vi "ITC503controlMonitor.vi"() -> ()   [LabVIEW 2019]
uses:
  Utility/ITC503/ITC503Monitor-Cluster.ctl
  Instrument_Setup.vi
  Global/Global Variables/Data_Display_global.vi
panel:
  out "error out":errorcluster
  in  "error in (no error)":errorcluster
  out "Path":path
  in  "stop":bool
  out "ITC503-Monitor":T1={"Temperatur (K)"=0.0, "Setpoint (K)"=0.0, "Rate (K/min)"=3.4572, "Heater (%)"=0.0, "NV (%)"=0.0, "Heater Manual"=FALSE, "NV Manual"=FALSE, "Go to Set"=FALSE, "Heater SP"=0.0, "Valid?"=FALSE, "Set Heater SP"=FALSE, "Set NV SP"=FALSE, "Heater (%) Display"=3.4572, "NV (%) Display"=3.4572, "NV Setpoint"=0.0, "Change Heater Status"=FALSE, "Change NV Status"=FALSE, "Sample 3"=0.0, "Sample 2"=0.0, "Sweep-State"=FALSE, "Set Auto PID"=FALSE, "Auto PID"=FALSE, "Stopp"=FALSE, "Setpoint-Sweep"=0.0, "Sample 1"=0.0, "Control Channel"=FALSE, "Channel 1"=FALSE, "Channel 2"=FALSE, "Channel 3"=FALSE} {"NV (%) Display" format="%4_5f"; "Heater (%) Display" format="%4_5f"; "NV (%)" scale=0.0..100.0; "Heater (%)" scale=0.0..100.0; "Rate (K/min)" format="%#4_5f"; "Setpoint (K)" format="%6_5f"}
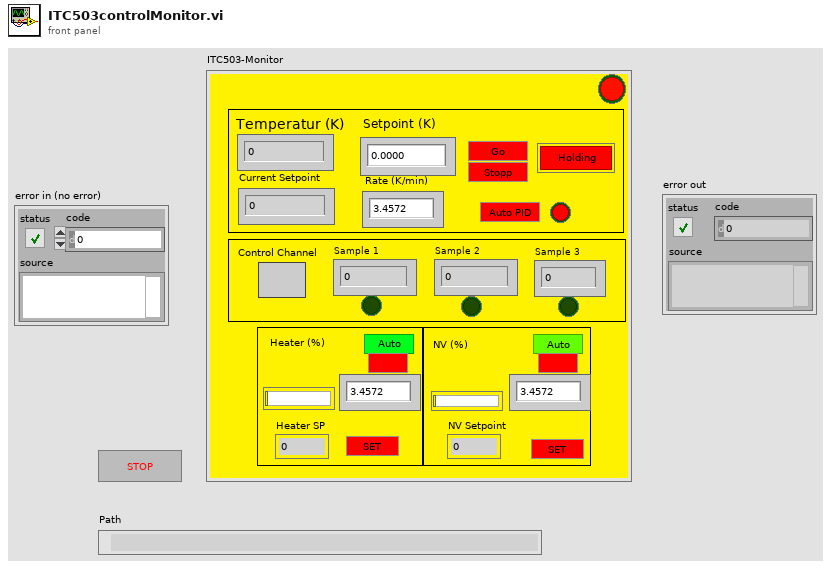
[diagram p1: front panel]
types:
  T1 = typedef "ITC503Monitor-Cluster.ctl" = cluster{"Temperatur (K)":dbl, "Setpoint (K)":dbl, "Rate (K/min)":dbl, "Heater (%)":dbl, "NV (%)":dbl, "Heater Manual":bool, "NV Manual":bool, "Go to Set":bool, "Heater SP":dbl, "Valid?":bool, "Set Heater SP":bool, "Set NV SP":bool, "Heater (%) Display":dbl, "NV (%) Display":dbl, "NV Setpoint":dbl, "Change Heater Status":bool, "Change NV Status":bool, "Sample 3":dbl, "Sample 2":dbl, "Sweep-State":bool, "Set Auto PID":bool, "Auto PID":bool, "Stopp":bool, "Setpoint-Sweep":dbl, "Sample 1":dbl, "Control Channel":bool, "Channel 1":bool, "Channel 2":bool, "Channel 3":bool}
  T2 = cluster{"Com Port":i32, "ISOBUS Address":i32, "GPIB Address":i16, "Communication":enum16{"RS232", "ISOBUS", "GPIB", "Gateway"}}
  T3 = typedef "OxfordAddress.ctl" = cluster{"Com Port":i32, "ISOBUS Address":i32, "GPIB Address":i16, "Communication":enum16{"RS232", "ISOBUS", "GPIB", "Gateway"}}
  T4 = enum32{"Bad", "Idle", "Run top level", "Running"}
  T5 = typedef "ITCIO.ctl" = cluster{"Com Port":i32, "ISOBUS Address":i32, "GPIB Address":i16, "Communication":enum16{"RS232", "ISOBUS", "GPIB", "Gateway"}}
  T6 = typedef "ITC503_control.ctl" = cluster{"Setpoint (K)":dbl, "Rate (K/min)":dbl, "Go to Set":bool, "Set Heater SP":bool, "Set NV SP":bool, "Change Heater Status":bool, "Change NV Status":bool, "Set Auto PID":bool, "Stopp":bool, "Control Channel":bool, "Heater SP":dbl, "NV Setpoint":dbl}
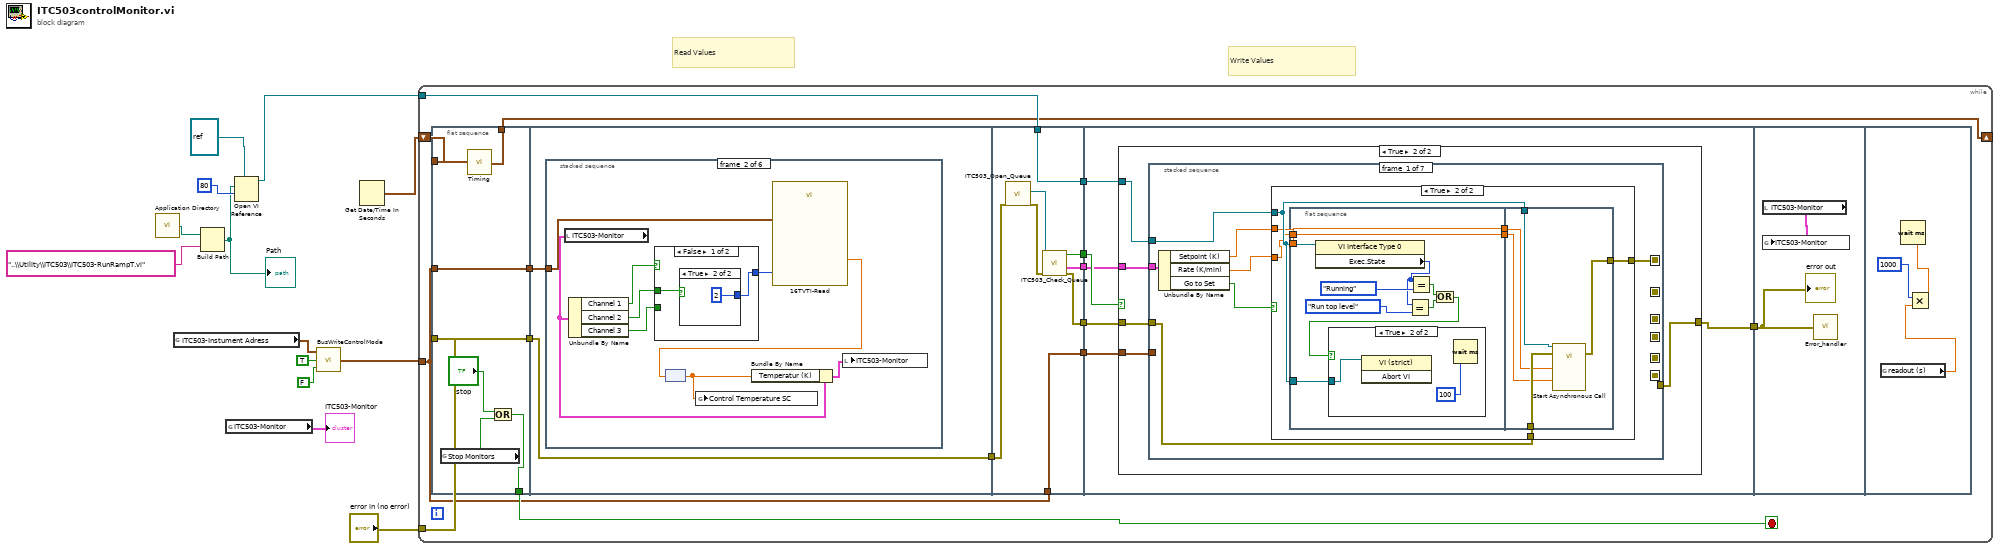
[diagram p0: block diagram]
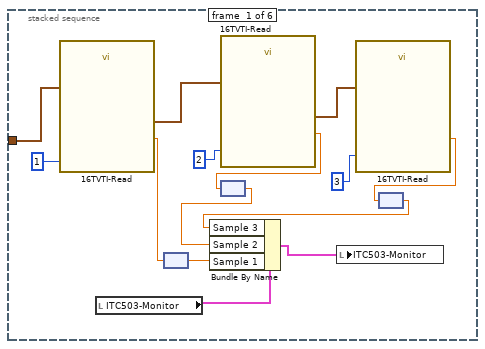
[diagram p2: hidden frame]
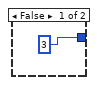
[diagram p3: hidden frame]
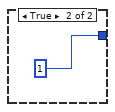
[diagram p4: hidden frame]
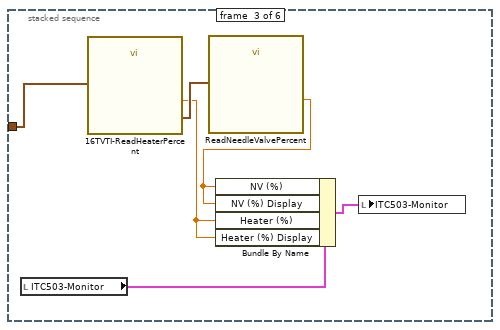
[diagram p5: hidden frame]
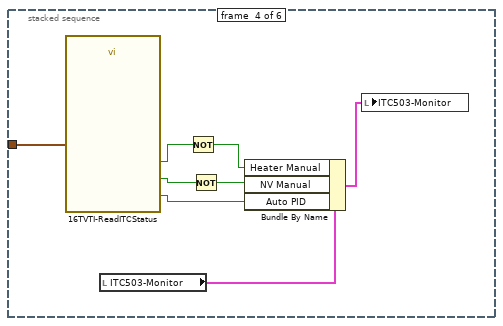
[diagram p6: hidden frame]
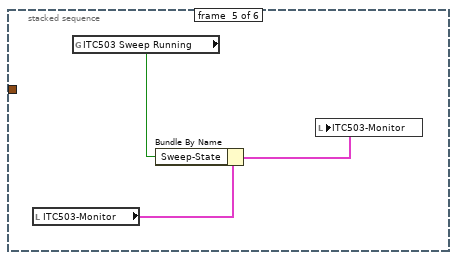
[diagram p7: hidden frame]
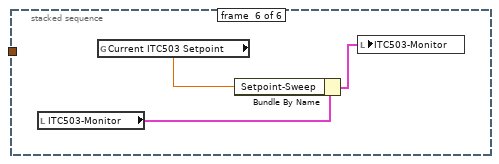
[diagram p8: hidden frame]
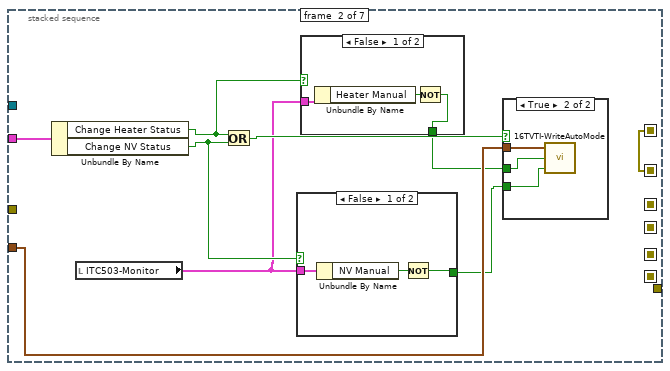
[diagram p12: hidden frame]
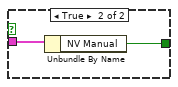
[diagram p14: hidden frame]
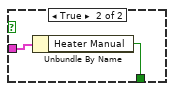
[diagram p15: hidden frame]
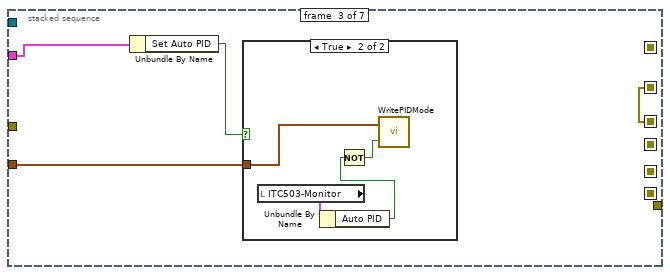
[diagram p16: hidden frame]
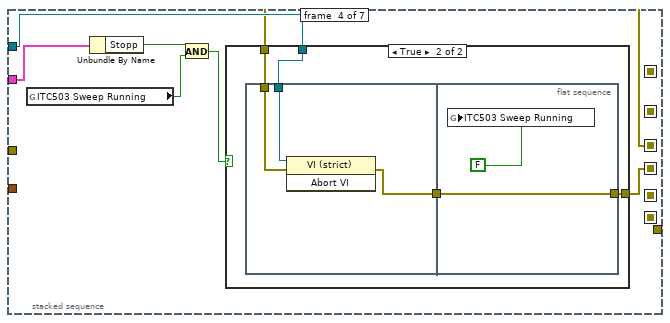
[diagram p18: hidden frame]
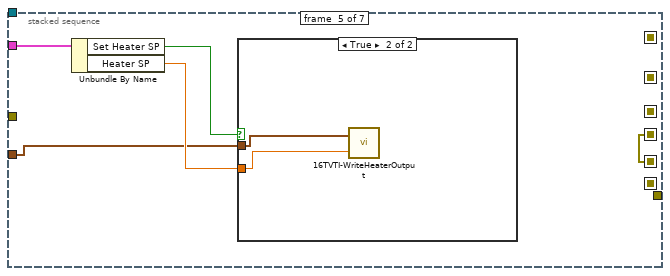
[diagram p20: hidden frame]
diagram:
  # "Write Values"
  # "Read Values"
  n1 = call <vilib>:"Application Directory.vi"() -> ("Application Directory"=w11:path)
  n2 = global read "Instrument_Setup.vi" "ITC503-Instument Adress"() -> (w8:T2)
  n3 = Build Path(base path=w11, name or relative path="..\\Utility\\ITC503\\ITC503-RunRampT.vi") -> (appended path=w9:path)
  "Path" <- w9
  n4 = global read "Data_Display_global.vi" "ITC503-Monitor"() -> (→"ITC503-Monitor":T1)
  n5 = Open VI Reference(type specifier VI Refnum (for type only)=refnum<vi> refnum, vi path=w9, options=80) -> (vi reference=w1:refnum<vi>)  [unwired: 3 in, 1 out]
  n6 = call "BusWriteControlMode.vi"("Locked"=FALSE, "Remote"=TRUE, "Address"=w8) -> ("Address(thru)"=w5:T3)
  n7 = Get Date/Time In Seconds() -> (seconds since 1Jan1904=w3:timestamp)
  n8 = while {
    tunnel: w5 -> [w16]
    shift-right: [w14] -> _
    shift-left: w3 -> [w27]
    tunnel: "error in (no error)" -> [w24]
    tunnel: w1 -> [w17]
    stop <- w28 stop-if-true
    n9 = flat-sequence {
      tunnel: [w33] -> w28
      tunnel: w27 -> [w32]
      tunnel: [w31] -> w14
      tunnel: w16 -> [w30]
      tunnel: [w30] -> w26
      tunnel: [w29] -> w25
      tunnel: w24 -> [w29]
      tunnel: w26 -> [w37]
      tunnel: w25 -> [w36]
      tunnel: [w36] -> w23
      tunnel: w23 -> [w93]
      tunnel: [w90] -> w22
      tunnel: [w89] -> w21
      tunnel: [w88] -> w20
      tunnel: [w87] -> w18
      tunnel: w17 -> [w87]
      tunnel: w16 -> [w86]
      tunnel: [w86] -> w15
      tunnel: w22 -> [w97]
      tunnel: w21 -> [w96]
      tunnel: w20 -> [w99]
      tunnel: [w98] -> w19
      tunnel: w18 -> [w95]
      tunnel: w15 -> [w94]
      tunnel: w19 -> [w215]
      frame #0 {
        n10 = global read "Data_Display_global.vi" "Stop Monitors"() -> (w34:bool)
        n11 = call "Timing.vi"("start time (s)"=w32) -> ("last reading (s)"=w31:timestamp)
        n12 = Or(x="stop", y=w34) -> (x .or. y?=w33:bool)
      }
      frame #1 {
        n13 = stacked-sequence {
          tunnel: w37 -> [w51 w60 w71 w79 _ _]
          frame #0 {
            n14 = call "16TVTI-Read.vi"("Channel"=1, "IO Info"=w51) -> ("Temperature"=w44:dbl[unit], "ITC IO Info"=w50:T5)  [unwired: 3 in, 1 out]
            n15 = local read "ITC503-Monitor"() -> (w45:T1)
            n16 = node(w44) -> (w43:dbl)
            n17 = call "16TVTI-Read.vi"("Channel"=2, "IO Info"=w50) -> ("Temperature"=w42:dbl[unit], "ITC IO Info"=w49:T5)  [unwired: 3 in, 1 out]
            n18 = node(w42) -> (w41:dbl)
            n19 = call "16TVTI-Read.vi"("Channel"=3, "IO Info"=w49) -> ("Temperature"=w40:dbl[unit])  [unwired: 3 in, 2 out]
            n20 = node(w40) -> (w39:dbl)
            n21 = Bundle By Name(cluster=w45, "Sample 3"=w39, "Sample 2"=w41, "Sample 1"=w43) -> (w38:T1)
            n22 = local write "ITC503-Monitor"(w38) -> ()
          }
          frame #1 {
            n23 = local read "ITC503-Monitor"() -> (w54:T1)
            n24 = Unbundle By Name(w54) -> ("Channel 1"=w59:bool, "Channel 2"=w57:bool, "Channel 3"=w56:bool)
            n25 = case shown="False" w59 {
              tunnel: [w61 1] -> w58
              tunnel: w57 -> [w62 _]
              tunnel: w56 -> [_ _]
              frame False {
                n26 = case shown="True" w62 {
                  tunnel: [3 2] -> w61
                  frame False {
                  }
                  frame True {
                  }
                }
              }
              frame True {
              }
            }
            n27 = call "16TVTI-Read.vi"("Channel"=w58, "IO Info"=w60) -> ("Temperature"=w55:dbl[unit])  [unwired: 3 in, 2 out]
            n28 = node(w55) -> (w52:dbl)
            n29 = global write "Data_Display_global.vi" "Control Temperature SC"(w52) -> ()
            n30 = Bundle By Name(cluster=w54, "Temperatur (K)"=w52) -> (w53:T1)
            n31 = local write "ITC503-Monitor"(w53) -> ()
          }
          frame #2 {
            n32 = local read "ITC503-Monitor"() -> (w69:T1)
            n33 = call "16TVTI-ReadHeaterPercent.vi"("ITC IO Info"=w71) -> ("Actual heater  %"=w67:dbl, "ITC IO Info"=w70:T5)  [unwired: 1 in]
            n34 = call "ReadNeedleValvePercent.vi"("IO Info"=w70) -> ("Actual Needle Valve  %"=w68:dbl)  [unwired: 1 in, 1 out]
            n35 = Bundle By Name(cluster=w69, "NV (%)"=w68, "NV (%) Display"=w68, "Heater (%)"=w67, "Heater (%) Display"=w67) -> (w66:T1)
            n36 = local write "ITC503-Monitor"(w66) -> ()
          }
          frame #3 {
            n37 = call "16TVTI-ReadITCStatus.vi"("ITC IO Info"=w79) -> ("Auto heat"=w74:bool, "Auto Needle Valve"=w75:bool, "Auto PID"=w77:bool)  [unwired: 4 in, 8 out]
            n38 = local read "ITC503-Monitor"() -> (w78:T1)
            n39 = Not(x=w74) -> (.not. x?=w73:bool)
            n40 = Not(x=w75) -> (.not. x?=w76:bool)
            n41 = Bundle By Name(cluster=w78, "Heater Manual"=w73, "NV Manual"=w76, "Auto PID"=w77) -> (w72:T1)
            n42 = local write "ITC503-Monitor"(w72) -> ()
          }
          frame #4 {
            n43 = local read "ITC503-Monitor"() -> (w82:T1)
            n44 = global read "Data_Display_global.vi" "ITC503 Sweep Running"() -> (w81:bool)
            n45 = Bundle By Name(cluster=w82, "Sweep-State"=w81) -> (w80:T1)
            n46 = local write "ITC503-Monitor"(w80) -> ()
          }
          frame #5 {
            n47 = local read "ITC503-Monitor"() -> (w85:T1)
            n48 = global read "Data_Display_global.vi" "Current ITC503 Setpoint"() -> (w84:dbl)
            n49 = Bundle By Name(cluster=w85, "Setpoint-Sweep"=w84) -> (w83:T1)
            n50 = local write "ITC503-Monitor"(w83) -> ()
          }
        }
      }
      frame #2 {
        n51 = call "ITC503_Open_Queue.vi"("error in (no error)"=w93) -> ("error out"=w91:errorcluster, "queue out"=w92:refnum<queue>)  [unwired: 9 in]
        n52 = call "ITC503_Check_Queue.vi"("error in (no error)"=w91, "queue"=w92) -> ("error out"=w88:errorcluster, "ITC503-Control"=w89:T6, "New Entries?"=w90:bool)  [unwired: 6 in]
      }
      frame #3 {
        n53 = case shown="True" w97 {
          tunnel: w99 -> [w100 w103]
          tunnel: [w100 w101] -> w98
          tunnel: w96 -> [_ w105]
          tunnel: w95 -> [_ w104]
          tunnel: w94 -> [_ w102]
          frame False {
          }
          frame True {
            n54 = stacked-sequence {
              seq-local: [w106 _ _ _ _ _ _] -> [_ w138 _ _ _ _ _]
              seq-local: [_ w138 _ _ _ _ _] -> [_ _ w162 _ _ _ _]
              seq-local: [_ _ w162 _ _ _ _] -> [_ _ _ w169 _ _ _]
              seq-local: [_ _ _ w168 _ _ _] -> [_ _ _ _ w185 _ _]
              seq-local: [_ _ _ _ w185 _ _] -> [_ _ _ _ _ w192 _]
              seq-local: [_ _ _ _ _ w192 _] -> [_ _ _ _ _ _ w200]
              tunnel: w105 -> [w112 w146 w163 w174 w189 w195 w203]
              tunnel: w104 -> [w108 _ _ w170 _ _ _]
              tunnel: w103 -> [w107 _ _ _ _ _ _]
              tunnel: w102 -> [_ w144 w160 _ w186 w196 w199]
              tunnel: [_ _ _ _ _ _ w200] -> w101
              frame #0 {
                n55 = Unbundle By Name(w112) -> ("Setpoint (K)"=w110:dbl, "Rate (K/min)"=w109:dbl, "Go to Set"=w111:bool)
                n56 = case shown="True" w111 {
                  tunnel: w110 -> [_ w118]
                  tunnel: w109 -> [_ w117]
                  tunnel: w108 -> [_ w120]
                  tunnel: w107 -> [w113 w115]
                  tunnel: [w113 w114] -> w106
                  frame False {
                  }
                  frame True {
                    n57 = flat-sequence {
                      tunnel: w120 -> [w130]
                      tunnel: w120 -> [w123]
                      tunnel: [w122] -> w119
                      tunnel: w118 -> [w122]
                      tunnel: w117 -> [w121]
                      tunnel: [w121] -> w116
                      tunnel: w120 -> [w137]
                      tunnel: w119 -> [w135]
                      tunnel: w116 -> [w134]
                      tunnel: w115 -> [w136]
                      tunnel: [w133] -> w114
                      frame #0 {
                        n58 = property class="VI Interface Type 0"(reference=w130) -> ("Exec.State"=w128:T4)  [unwired: 1 in, 2 out]
                        n59 = Equal?(x=w128, y=T4."Run top level" ("LS 370 Monitor 2")) -> (x = y?=w125:bool)
                        n60 = Equal?(x=w128, y=T4."Running" ("LS 370 Monitor 2")) -> (x = y?=w126:bool)
                        n61 = Or(x=w126, y=w125) -> (x .or. y?=w124:bool)
                        n62 = case shown="True" w124 {
                          tunnel: w123 -> [_ w132]
                          frame False {
                          }
                          frame True {
                            n63 = invoke class="VI (strict)" method="Abort VI"(reference=w132) -> ()  [unwired: 2 in, 3 out]
                            n64 = Wait (ms)(milliseconds to wait=100) -> ()  [unwired: 1 out]
                          }
                        }
                      }
                      frame #1 {
                        n65 = call-by-ref "Start Asynchronous Call"(reference=w137, error in=w136, "Rate (K/min)"=w134, "Final T (K)"=w135) -> (error out=w133:errorcluster)  [unwired: 2 out]
                      }
                    }
                  }
                }
              }
              frame #1 {
                n66 = Unbundle By Name(w146) -> ("Change Heater Status"=w142:bool, "Change NV Status"=w143:bool)
                n67 = local read "ITC503-Monitor"() -> (w141:T1)
                n68 = Or(x=w142, y=w143) -> (x .or. y?=w145:bool)
                n69 = case shown="False" w143 {
                  tunnel: w141 -> [w152 w154]
                  tunnel: [w151 w153] -> w139
                  frame False {
                    n70 = Unbundle By Name(w152) -> ("NV Manual"=w150:bool)
                    n71 = Not(x=w150) -> (.not. x?=w151:bool)
                  }
                  frame True {
                    n72 = Unbundle By Name(w154) -> ("NV Manual"=w153:bool)
                  }
                }
                n73 = case shown="False" w142 {
                  tunnel: w141 -> [w157 w159]
                  tunnel: [w155 w158] -> w140
                  frame False {
                    n74 = Unbundle By Name(w157) -> ("Heater Manual"=w156:bool)
                    n75 = Not(x=w156) -> (.not. x?=w155:bool)
                  }
                  frame True {
                    n76 = Unbundle By Name(w159) -> ("Heater Manual"=w158:bool)
                  }
                }
                n77 = case shown="True" w145 {
                  tunnel: w144 -> [_ w149]
                  tunnel: w140 -> [_ w148]
                  tunnel: w139 -> [_ w147]
                  frame False {
                  }
                  frame True {
                    n78 = call "16TVTI-WriteAutoMode.vi"("Auto Needle Valve"=w147, "Auto Heat"=w148, "Instrument address"=w149) -> ()  [unwired: 1 out]
                  }
                }
              }
              frame #2 {
                n79 = Unbundle By Name(w163) -> ("Set Auto PID"=w161:bool)
                n80 = case shown="True" w161 {
                  tunnel: w160 -> [_ w167]
                  frame False {
                  }
                  frame True {
                    n81 = local read "ITC503-Monitor"() -> (w166:T1)
                    n82 = Unbundle By Name(w166) -> ("Auto PID"=w164:bool)
                    n83 = Not(x=w164) -> (.not. x?=w165:bool)
                    n84 = call "WritePIDMode.vi"("Auto PID"=w165, "Instrument address"=w167) -> ()  [unwired: 1 in, 1 out]
                  }
                }
              }
              frame #3 {
                n85 = global read "Data_Display_global.vi" "ITC503 Sweep Running"() -> (w172:bool)
                n86 = Unbundle By Name(w174) -> ("Stopp"=w173:bool)
                n87 = And(x=w173, y=w172) -> (x .and. y?=w171:bool)
                n88 = case shown="True" w171 {
                  tunnel: w170 -> [_ w179]
                  tunnel: w169 -> [w175 w178]
                  tunnel: [w175 w176] -> w168
                  frame False {
                  }
                  frame True {
                    n89 = flat-sequence {
                      tunnel: w179 -> [w182]
                      tunnel: w178 -> [w181]
                      tunnel: [w180] -> w177
                      tunnel: [w183] -> w176
                      tunnel: w177 -> [w183]
                      frame #0 {
                        n90 = invoke class="VI (strict)" method="Abort VI"(reference=w182, error in=w181) -> (error out=w180:errorcluster)  [unwired: 1 in, 2 out]
                      }
                      frame #1 {
                        n91 = global write "Data_Display_global.vi" "ITC503 Sweep Running"(FALSE) -> ()
                      }
                    }
                  }
                }
              }
              frame #4 {
                n92 = Unbundle By Name(w189) -> ("Set Heater SP"=w188:bool, "Heater SP"=w187:dbl)
                n93 = case shown="True" w188 {
                  tunnel: w187 -> [_ w191]
                  tunnel: w186 -> [_ w190]
                  frame False {
                  }
                  frame True {
                    n94 = call "16TVTI-WriteHeaterOutput.vi"("Heater Output (%)"=w191, "ITC IO Info"=w190) -> ()  [unwired: 1 in, 1 out]
                  }
                }
              }
              frame #5 {
                n95 = Unbundle By Name(w195) -> ("Set NV SP"=w194:bool, "NV Setpoint"=w193:dbl)
                n96 = case shown="True" w194 {
                  tunnel: w196 -> [_ w198]
                  tunnel: w193 -> [_ w197]
                  frame False {
                  }
                  frame True {
                    n97 = call "16TVTI-WriteNeedleValveOutput.vi"("Needle Valve Output (%"=w197, "ITC IO Info"=w198) -> ()  [unwired: 1 in, 1 out]
                  }
                }
              }
              frame #6 {
                n98 = Unbundle By Name(w203) -> ("Control Channel"=w202:bool)
                n99 = local read "ITC503-Monitor"() -> (w201:T1)
                n100 = case shown="True" w202 {
                  tunnel: w201 -> [_ w206]
                  tunnel: w199 -> [_ w204]
                  frame False {
                  }
                  frame True {
                    n101 = Unbundle By Name(w206) -> ("Channel 1"=w207:bool)
                    n102 = case shown="False" w207 {
                      tunnel: [w208 2] -> w205
                      tunnel: w206 -> [w210 _]
                      frame False {
                        n103 = Unbundle By Name(w210) -> ("Channel 2"=w209:bool)
                        n104 = case shown="False" w209 {
                          tunnel: [1 3] -> w208
                          frame False {
                          }
                          frame True {
                          }
                        }
                      }
                      frame True {
                      }
                    }
                    n105 = call "writeITC503control_channel.vi"("Control Channel"=w205, "ITC IO Info 2"=w204) -> ()  [unwired: 3 in, 1 out]
                  }
                }
              }
            }
          }
        }
      }
      frame #4 {
        n106 = local read "ITC503-Monitor"() -> (w214:T1)
        n107 = global write "Data_Display_global.vi" "ITC503-Monitor"(w214) -> ()
        n108 = call "Error_handler.vi"("error constant"=w215) -> ()
        "error out" <- w215
      }
      frame #5 {
        n109 = global read "Instrument_Setup.vi" "readout (s)"() -> (w218:dbl)
        n110 = Multiply(x=1000, y=w218) -> (x*y=w217:dbl)
        n111 = Wait (ms)(milliseconds to wait=w217) -> ()  [unwired: 1 out]
      }
    }
  }
